vi "A4_Verificador_Info.vi"() -> ()   [LabVIEW 2025]
panel:
  in  "Table Control":string[][](table)
  out "Nombre confirmado":string
  in  "Contraseña":string
  in  "Nombre":string
  out "Boolean":bool
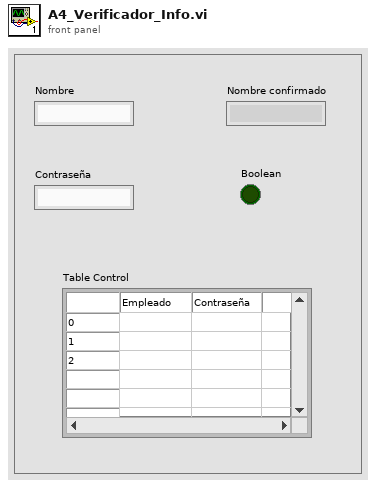
[diagram p1: front panel]
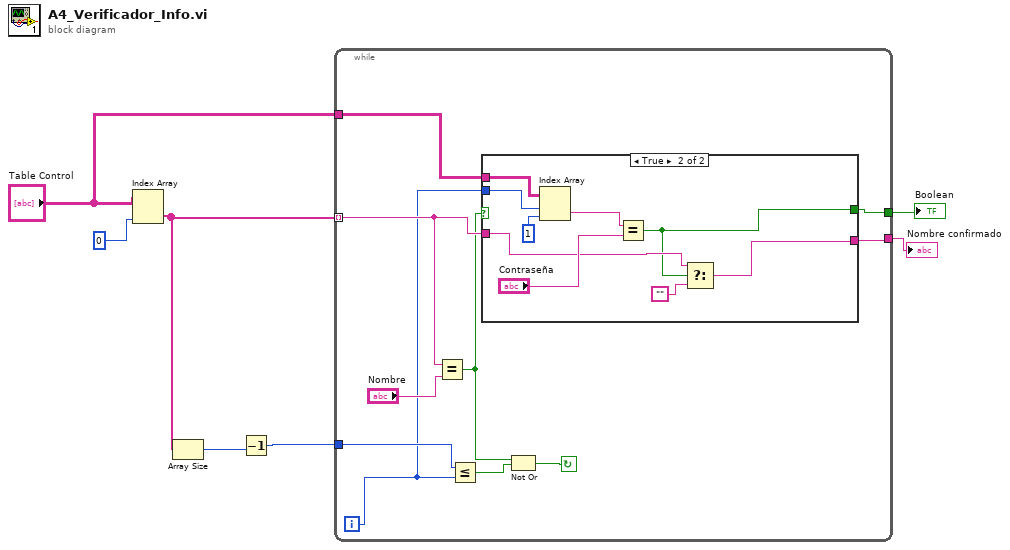
[diagram p0: block diagram]
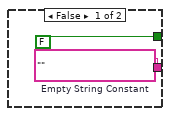
[diagram p2: hidden frame]
diagram:
  n1 = Index Array "Index Array"(array="Table Control", index (col)=0 ("index")) -> (element=w4:string[])  [unwired: 1 in]
  n2 = Array Size(array=w4) -> (size(s)=w7:i32)
  n3 = Decrement(x=w7) -> (x-1=w6:i32)
  n4 = while {
    tunnel: w6 -> [w14]
    tunnel: "Table Control" -> [w17]
    tunnel: w4 -> [w15] mode=indexing
    tunnel: [w9] -> w3
    tunnel: [w8] -> w2
    i -> [w13]
    stop <- w10 continue-if-true
    n5 = Equal?(x=w15, y="Nombre") -> (x = y?=w11:bool)
    n6 = Less Or Equal?(x=w14, y=w13) -> (x <= y?=w12:bool)
    n7 = case shown="True" w11 {
      tunnel: w17 -> [_ w28]
      tunnel: w15 -> [_ w23]
      tunnel: w13 -> [_ w27]
      tunnel: [w18 w22] -> w9
      tunnel: [FALSE w21] -> w8
      frame False {
        w18 = ""  # Empty String Constant
      }
      frame True {
        n8 = Index Array(array=w28, index (row)=w27, index (col)=1) -> (element=w25:string)
        n9 = Equal?(x=w25, y="Contraseña") -> (x = y?=w21:bool)
        n10 = Select(t=w23, s=w21, f="") -> (s? t:f=w22:string)
      }
    }
    n11 = Not Or(1:w12, 2:w11) -> (0:w10:bool)
  }
  "Nombre confirmado" <- w3
  "Boolean" <- w2
